vi "Lines LoadArrayOfSessions.vi"(8 "error in (no error)":errorcluster, 10 "regular expression":string, 11 "Lines":string[](array[string])) -> (0 "error out":errorcluster, 1 "Matched Sessions":string[](array[string]), 2 "String Config Group":cluster{"name":string, "cfg":string}[](array[cluster]), 3 "Config Text List out":string[](array[string]))   [LabVIEW 2012]
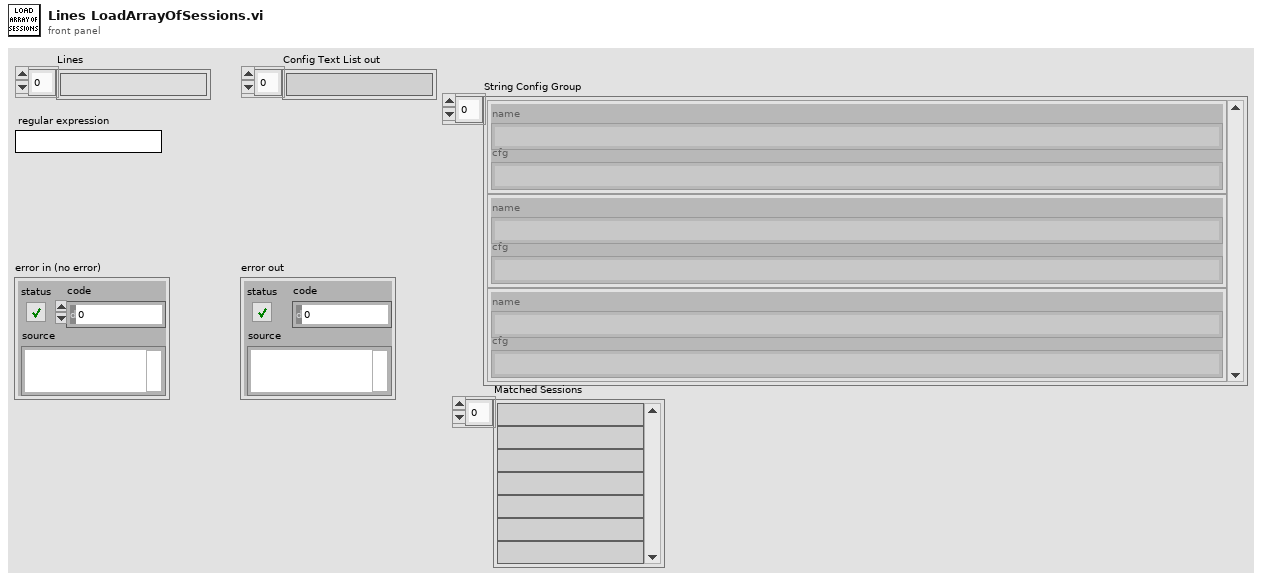
[diagram p1: front panel]
types:
  T1 = cluster{"name":string, "trimmed string":string}[]
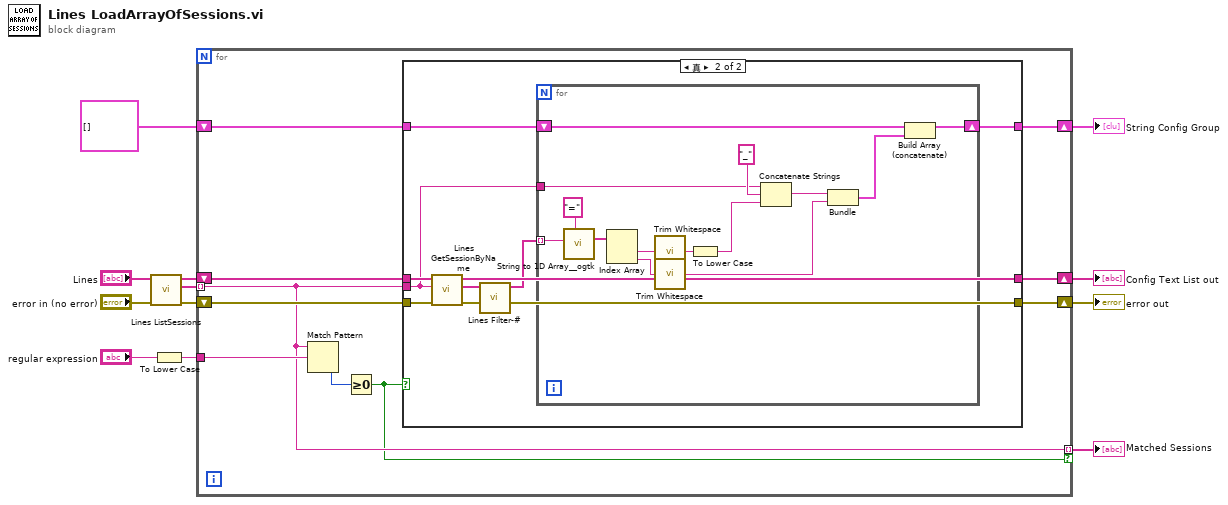
[diagram p0: block diagram]
diagram:
  n1 = call "Lines ListSessions.vi"("error in (no error)"="error in (no error)", "Config Text List"="Lines") -> ("error out"=w6:errorcluster, "Sessions"=w9:string[], "Config Text List out"=w7:string[])  [unwired: 7 in]
  n2 = To Lower Case(string="regular expression") -> (all lower case string=w12:string)
  n3 = for {
    shift-right: [w20] -> w8
    shift-left: w7 -> [w21]
    tunnel: w9 -> [w14] mode=indexing
    shift-right: [w18] -> w10
    shift-left: w6 -> [w22]
    tunnel: w12 -> [w17]
    shift-right: [w16] -> w2
    shift-left: cluster{"name":string, "cfg":string}[] [] ("String Config Group") -> [w15]
    tunnel: [w14] -> w1 mode=indexing if=w13
    n4 = Match Pattern(string=w14, regular expression=w17) -> (offset past match=w19:i32)  [unwired: 1 in, 3 out]
    n5 = Greater Or Equal To 0?(x=w19) -> (x >= 0?=w13:bool)
    n6 = case shown="真" w13 {
      tunnel: w22 -> [w24 w34]
      tunnel: w21 -> [w25 w32]
      tunnel: [w25 w31] -> w20
      tunnel: w14 -> [_ w29]
      tunnel: [w24 w28] -> w18
      tunnel: [w23 w27] -> w16
      tunnel: w15 -> [w23 w26]
      frame False {
      }
      frame True {
        n7 = call "Lines GetSessionByName.vi"("error in (no error)"=w34, "[] Session Name"=w29, "Config Text List"=w32) -> ("error out"=w35:errorcluster, "Session"=w33:string[], "Config Text List out"=w31:string[])  [unwired: 6 in]
        n8 = call "Lines Filter-#.vi"("error in (no error)"=w35, "Lines"=w33) -> ("error out"=w28:errorcluster, "Config Text List"=w30:string[])  [unwired: 8 in]
        n9 = for {
          tunnel: w30 -> [w45] mode=indexing
          tunnel: w29 -> [w43]
          shift-right: [w40] -> w27
          shift-left: w26 -> [w41]
          n10 = call <userlib>:"String to 1D Array__ogtk.vi"("delimiter (Tab)"="=", "string"=w45) -> ("Array of Strings"=w47:string[])  [unwired: 9 in]
          n11 = Index Array(array=w47) -> (element #1=w48:string, element #2=w49:string)  [unwired: 2 in]
          n12 = call <vilib>:"Trim Whitespace.vi"("string"=w48) -> ("trimmed string"=w42:string)  [unwired: 1 in]
          n13 = call <vilib>:"Trim Whitespace.vi"("string"=w49) -> ("trimmed string"=w38:string)  [unwired: 1 in]
          n14 = To Lower Case(string=w42) -> (all lower case string=w36:string)
          n15 = Concatenate Strings(w43, "_" ("delimiter (Tab)"), w36) -> (w39:string)
          n16 = Bundle(w39, "trimmed string"=w38) -> (w37:cluster{string, "trimmed string":string})  [unwired: 1 in]
          n17 = Build Array (concatenate)(w41, w37) -> (w40:T1)
        }
      }
    }
  }
  "error out" <- w10
  "Config Text List out" <- w8
  "String Config Group" <- w2
  "Matched Sessions" <- w1
